vi "writeSettingsFile4ch.vi"(4 "delimiter (,)":string=",", 6 "message (overrides settings)":string, 7 "timestamp (current)":timestamp, 8 "error in (no error)":errorcluster, 9 "old settings":T3={"sampling"=1000, "coincidence_window"=10, "delay_A"=0, "delay_B"=0, "delay_C"=0, "delay_D"=0, "sleep_A"=0, "sleep_B"=0, "sleep_C"=0, "sleep_D"=0, "config_multiple_1"=0} {"config_multiple_1" items=["ABC"=224, "ABD"=208, "ACD"=176, "BCD"=112, "ABCD"=240]; "sleep_D" max=100 step=5; "sleep_C" max=100 step=5; "sleep_B" max=100 step=5; "sleep_A" max=100 step=5; "delay_D" max=100 step=5; "delay_C" max=100 step=5; "delay_B" max=100 step=5; "delay_A" max=100 step=5; "coincidence_window" min=5 max=10000 step=5; "sampling" items=["1ms"=1, "2ms"=2, "3ms"=3, "4ms"=4, "5ms"=5, "6ms"=6, "7ms"=7, "8ms"=8, "9ms"=9, "10ms"=10, "11ms"=11, "12ms"=12, "13ms"=13, "14ms"=14, "15ms"=15, "16ms"=16, "17ms"=17, "18ms"=18, "19ms"=19, "20ms"=20, "21ms"=21, "22ms"=22, "23ms"=23, "24ms"=24, "25ms"=25, "26ms"=26, "27ms"=27, "28ms"=28, "29ms"=29, "30ms"=30, "31ms"=31, "32ms"=32, "33ms"=33, "34ms"=34, "35ms"=35, "36ms"=36, "37ms"=37, "38ms"=38, "39ms"=39, "40ms"=40, "41ms"=41, "42ms"=42, "43ms"=43, "44ms"=44, "45ms"=45, "46ms"=46, "47ms"=47, "48ms"=48, "49ms"=49, "50ms"=50, "51ms"=51, "52ms"=52, "53ms"=53, "54ms"=54, "55ms"=55, "56ms"=56, "57ms"=57, "58ms"=58, "59ms"=59, "60ms"=60, "61ms"=61, "62ms"=62, "63ms"=63, "64ms"=64, "65ms"=65, "66ms"=66, "67ms"=67, "68ms"=68, "69ms"=69, "70ms"=70, "71ms"=71, "72ms"=72, "73ms"=73, "74ms"=74, "75ms"=75, "76ms"=76, "77ms"=77, "78ms"=78, "79ms"=79, "80ms"=80, "81ms"=81, "82ms"=82, "83ms"=83, "84ms"=84, "85ms"=85, "86ms"=86, "87ms"=87, "88ms"=88, "89ms"=89, "90ms"=90, "91ms"=91, "92ms"=92, "93ms"=93, "94ms"=94, "95ms"=95, "96ms"=96, "97ms"=97, "98ms"=98, "99ms"=99, "100ms"=100, "110ms"=110, "120ms"=120, "130ms"=130, "140ms"=140, "150ms"=150, "160ms"=160, "170ms"=170, "180ms"=180, "190ms"=190, "200ms"=200, "210ms"=210, "220ms"=220, "230ms"=230, "240ms"=240, "250ms"=250, "260ms"=260, "270ms"=270, "280ms"=280, "290ms"=290, "300ms"=300, "310ms"=310, "320ms"=320, "330ms"=330, "340ms"=340, "350ms"=350, "360ms"=360, "370ms"=370, "380ms"=380, "390ms"=390, "400ms"=400, "410ms"=410, "420ms"=420, "430ms"=430, "440ms"=440, "450ms"=450, "460ms"=460, "470ms"=470, "480ms"=480, "490ms"=490, "500ms"=500, "510ms"=510, "520ms"=520, "530ms"=530, "540ms"=540, "550ms"=550, "560ms"=560, "570ms"=570, "580ms"=580, "590ms"=590, "600ms"=600, "610ms"=610, "620ms"=620, "630ms"=630, "640ms"=640, "650ms"=650, "660ms"=660, "670ms"=670, "680ms"=680, "690ms"=690, "700ms"=700, "710ms"=710, "720ms"=720, "730ms"=730, "740ms"=740, "750ms"=750, "760ms"=760, "770ms"=770, "780ms"=780, "790ms"=790, "800ms"=800, "810ms"=810, "820ms"=820, "830ms"=830, "840ms"=840, "850ms"=850, "860ms"=860, "870ms"=870, "880ms"=880, "890ms"=890, "900ms"=900, "910ms"=910, "920ms"=920, "930ms"=930, "940ms"=940, "950ms"=950, "960ms"=960, "970ms"=970, "980ms"=980, "990ms"=990, "1,0s"=1000, "1,1s"=1100, "1,2s"=1200, "1,3s"=1300, "1,4s"=1400, "1,5s"=1500, "1,6s"=1600, "1,7s"=1700, "1,8s"=1800, "1,9s"=1900, "2,0s"=2000, "2,1s"=2100, "2,2s"=2200, "2,3s"=2300, "2,4s"=2400, "2,5s"=2500, "2,6s"=2600, "2,7s"=2700, "2,8s"=2800, "2,9s"=2900, "3,0s"=3000, "3,1s"=3100, "3,2s"=3200, "3,3s"=3300, "3,4s"=3400, "3,5s"=3500, "3,6s"=3600, "3,7s"=3700, "3,8s"=3800, "3,9s"=3900, "4,0s"=4000, "4,1s"=4100, "4,2s"=4200, "4,3s"=4300, "4,4s"=4400, "4,5s"=4500, "4,6s"=4600, "4,7s"=4700, "4,8s"=4800, "4,9s"=4900, "5,0s"=5000, "5,1s"=5100, "5,2s"=5200, "5,3s"=5300, "5,4s"=5400, "5,5s"=5500, "5,6s"=5600, "5,7s"=5700, "5,8s"=5800, "5,9s"=5900, "6,0s"=6000, "6,1s"=6100, "6,2s"=6200, "6,3s"=6300, "6,4s"=6400, "6,5s"=6500, "6,6s"=6600, "6,7s"=6700, "6,8s"=6800, "6,9s"=6900, "7,0s"=7000, "7,1s"=7100, "7,2s"=7200, "7,3s"=7300, "7,4s"=7400, "7,5s"=7500, "7,6s"=7600, "7,7s"=7700, "7,8s"=7800, "7,9s"=7900, "8,0s"=8000, "8,1s"=8100, "8,2s"=8200, "8,3s"=8300, "8,4s"=8400, "8,5s"=8500, "8,6s"=8600, "8,7s"=8700, "8,8s"=8800, "8,9s"=8900, "9,0s"=9000, "9,1s"=9100, "9,2s"=9200, "9,3s"=9300, "9,4s"=9400, "9,5s"=9500, "9,6s"=9600, "9,7s"=9700, "9,8s"=9800, "9,9s"=9900, "10s"=10000, "11s"=11000, "12s"=12000, "13s"=13000, "14s"=14000, "15s"=15000, "16s"=16000, "17s"=17000, "18s"=18000, "19s"=19000, "20s"=20000, "21s"=21000, "22s"=22000, "23s"=23000, "24s"=24000, "25s"=25000, "26s"=26000, "27s"=27000, "28s"=28000, "29s"=29000, "30s"=30000, "31s"=31000, "32s"=32000, "33s"=33000, "34s"=34000, "35s"=35000, "36s"=36000, "37s"=37000, "38s"=38000, "39s"=39000, "40s"=40000, "41s"=41000, "42s"=42000, "43s"=43000, "44s"=44000, "45s"=45000, "46s"=46000, "47s"=47000, "48s"=48000, "49s"=49000, "50s"=50000, "51s"=51000, "52s"=52000, "53s"=53000, "54s"=54000, "55s"=55000, "56s"=56000, "57s"=57000, "58s"=58000, "59s"=59000, "60s"=60000, "61s"=61000, "62s"=62000, "63s"=63000, "64s"=64000, "65s"=65000, "66s"=66000, "67s"=67000, "68s"=68000, "69s"=69000, "70s"=70000, "71s"=71000, "72s"=72000, "73s"=73000, "74s"=74000, "75s"=75000, "76s"=76000, "77s"=77000, "78s"=78000, "79s"=79000, "80s"=80000, "81s"=81000, "82s"=82000, "83s"=83000, "84s"=84000, "85s"=85000, "86s"=86000, "87s"=87000, "88s"=88000, "89s"=89000, "90s"=90000, "91s"=91000, "92s"=92000, "93s"=93000, "94s"=94000, "95s"=95000, "96s"=96000, "97s"=97000, "98s"=98000, "99s"=99000, "100s"=100000, "110s"=110000, "120s"=120000, "130s"=130000, "140s"=140000, "150s"=150000, "160s"=160000, "170s"=170000, "180s"=180000, "190s"=190000, "200s"=200000, "210s"=210000, "220s"=220000, "230s"=230000, "240s"=240000, "250s"=250000, "260s"=260000, "270s"=270000, "280s"=280000, "290s"=290000, "300s"=300000, "310s"=310000, "320s"=320000, "330s"=330000, "340s"=340000, "350s"=350000, "360s"=360000, "370s"=370000, "380s"=380000, "390s"=390000, "400s"=400000, "410s"=410000, "420s"=420000, "430s"=430000, "440s"=440000, "450s"=450000, "460s"=460000, "470s"=470000, "480s"=480000, "490s"=490000, "500s"=500000, "510s"=510000, "520s"=520000, "530s"=530000, "540s"=540000, "550s"=550000, "560s"=560000, "570s"=570000, "580s"=580000, "590s"=590000, "600s"=600000, "610s"=610000, "620s"=620000, "630s"=630000, "640s"=640000, "650s"=650000, "660s"=660000, "670s"=670000, "680s"=680000, "690s"=690000, "700s"=700000, "710s"=710000, "720s"=720000, "730s"=730000, "740s"=740000, "750s"=750000, "760s"=760000, "770s"=770000, "780s"=780000, "790s"=790000, "800s"=800000, "810s"=810000, "820s"=820000, "830s"=830000, "840s"=840000, "850s"=850000, "860s"=860000, "870s"=870000, "880s"=880000, "890s"=890000, "900s"=900000, "910s"=910000, "920s"=920000, "930s"=930000, "940s"=940000, "950s"=950000, "960s"=960000, "970s"=970000, "980s"=980000, "990s"=990000, "1000s"=1000000]}, 10 "new settings":T3={"sampling"=1000, "coincidence_window"=10, "delay_A"=0, "delay_B"=0, "delay_C"=0, "delay_D"=0, "sleep_A"=0, "sleep_B"=0, "sleep_C"=0, "sleep_D"=0, "config_multiple_1"=0} {"config_multiple_1" items=["ABC"=224, "ABD"=208, "ACD"=176, "BCD"=112, "ABCD"=240]; "sleep_D" max=100 step=5; "sleep_C" max=100 step=5; "sleep_B" max=100 step=5; "sleep_A" max=100 step=5; "delay_D" max=100 step=5; "delay_C" max=100 step=5; "delay_B" max=100 step=5; "delay_A" max=100 step=5; "coincidence_window" min=5 max=10000 step=5; "sampling" items=["1ms"=1, "2ms"=2, "3ms"=3, "4ms"=4, "5ms"=5, "6ms"=6, "7ms"=7, "8ms"=8, "9ms"=9, "10ms"=10, "11ms"=11, "12ms"=12, "13ms"=13, "14ms"=14, "15ms"=15, "16ms"=16, "17ms"=17, "18ms"=18, "19ms"=19, "20ms"=20, "21ms"=21, "22ms"=22, "23ms"=23, "24ms"=24, "25ms"=25, "26ms"=26, "27ms"=27, "28ms"=28, "29ms"=29, "30ms"=30, "31ms"=31, "32ms"=32, "33ms"=33, "34ms"=34, "35ms"=35, "36ms"=36, "37ms"=37, "38ms"=38, "39ms"=39, "40ms"=40, "41ms"=41, "42ms"=42, "43ms"=43, "44ms"=44, "45ms"=45, "46ms"=46, "47ms"=47, "48ms"=48, "49ms"=49, "50ms"=50, "51ms"=51, "52ms"=52, "53ms"=53, "54ms"=54, "55ms"=55, "56ms"=56, "57ms"=57, "58ms"=58, "59ms"=59, "60ms"=60, "61ms"=61, "62ms"=62, "63ms"=63, "64ms"=64, "65ms"=65, "66ms"=66, "67ms"=67, "68ms"=68, "69ms"=69, "70ms"=70, "71ms"=71, "72ms"=72, "73ms"=73, "74ms"=74, "75ms"=75, "76ms"=76, "77ms"=77, "78ms"=78, "79ms"=79, "80ms"=80, "81ms"=81, "82ms"=82, "83ms"=83, "84ms"=84, "85ms"=85, "86ms"=86, "87ms"=87, "88ms"=88, "89ms"=89, "90ms"=90, "91ms"=91, "92ms"=92, "93ms"=93, "94ms"=94, "95ms"=95, "96ms"=96, "97ms"=97, "98ms"=98, "99ms"=99, "100ms"=100, "110ms"=110, "120ms"=120, "130ms"=130, "140ms"=140, "150ms"=150, "160ms"=160, "170ms"=170, "180ms"=180, "190ms"=190, "200ms"=200, "210ms"=210, "220ms"=220, "230ms"=230, "240ms"=240, "250ms"=250, "260ms"=260, "270ms"=270, "280ms"=280, "290ms"=290, "300ms"=300, "310ms"=310, "320ms"=320, "330ms"=330, "340ms"=340, "350ms"=350, "360ms"=360, "370ms"=370, "380ms"=380, "390ms"=390, "400ms"=400, "410ms"=410, "420ms"=420, "430ms"=430, "440ms"=440, "450ms"=450, "460ms"=460, "470ms"=470, "480ms"=480, "490ms"=490, "500ms"=500, "510ms"=510, "520ms"=520, "530ms"=530, "540ms"=540, "550ms"=550, "560ms"=560, "570ms"=570, "580ms"=580, "590ms"=590, "600ms"=600, "610ms"=610, "620ms"=620, "630ms"=630, "640ms"=640, "650ms"=650, "660ms"=660, "670ms"=670, "680ms"=680, "690ms"=690, "700ms"=700, "710ms"=710, "720ms"=720, "730ms"=730, "740ms"=740, "750ms"=750, "760ms"=760, "770ms"=770, "780ms"=780, "790ms"=790, "800ms"=800, "810ms"=810, "820ms"=820, "830ms"=830, "840ms"=840, "850ms"=850, "860ms"=860, "870ms"=870, "880ms"=880, "890ms"=890, "900ms"=900, "910ms"=910, "920ms"=920, "930ms"=930, "940ms"=940, "950ms"=950, "960ms"=960, "970ms"=970, "980ms"=980, "990ms"=990, "1,0s"=1000, "1,1s"=1100, "1,2s"=1200, "1,3s"=1300, "1,4s"=1400, "1,5s"=1500, "1,6s"=1600, "1,7s"=1700, "1,8s"=1800, "1,9s"=1900, "2,0s"=2000, "2,1s"=2100, "2,2s"=2200, "2,3s"=2300, "2,4s"=2400, "2,5s"=2500, "2,6s"=2600, "2,7s"=2700, "2,8s"=2800, "2,9s"=2900, "3,0s"=3000, "3,1s"=3100, "3,2s"=3200, "3,3s"=3300, "3,4s"=3400, "3,5s"=3500, "3,6s"=3600, "3,7s"=3700, "3,8s"=3800, "3,9s"=3900, "4,0s"=4000, "4,1s"=4100, "4,2s"=4200, "4,3s"=4300, "4,4s"=4400, "4,5s"=4500, "4,6s"=4600, "4,7s"=4700, "4,8s"=4800, "4,9s"=4900, "5,0s"=5000, "5,1s"=5100, "5,2s"=5200, "5,3s"=5300, "5,4s"=5400, "5,5s"=5500, "5,6s"=5600, "5,7s"=5700, "5,8s"=5800, "5,9s"=5900, "6,0s"=6000, "6,1s"=6100, "6,2s"=6200, "6,3s"=6300, "6,4s"=6400, "6,5s"=6500, "6,6s"=6600, "6,7s"=6700, "6,8s"=6800, "6,9s"=6900, "7,0s"=7000, "7,1s"=7100, "7,2s"=7200, "7,3s"=7300, "7,4s"=7400, "7,5s"=7500, "7,6s"=7600, "7,7s"=7700, "7,8s"=7800, "7,9s"=7900, "8,0s"=8000, "8,1s"=8100, "8,2s"=8200, "8,3s"=8300, "8,4s"=8400, "8,5s"=8500, "8,6s"=8600, "8,7s"=8700, "8,8s"=8800, "8,9s"=8900, "9,0s"=9000, "9,1s"=9100, "9,2s"=9200, "9,3s"=9300, "9,4s"=9400, "9,5s"=9500, "9,6s"=9600, "9,7s"=9700, "9,8s"=9800, "9,9s"=9900, "10s"=10000, "11s"=11000, "12s"=12000, "13s"=13000, "14s"=14000, "15s"=15000, "16s"=16000, "17s"=17000, "18s"=18000, "19s"=19000, "20s"=20000, "21s"=21000, "22s"=22000, "23s"=23000, "24s"=24000, "25s"=25000, "26s"=26000, "27s"=27000, "28s"=28000, "29s"=29000, "30s"=30000, "31s"=31000, "32s"=32000, "33s"=33000, "34s"=34000, "35s"=35000, "36s"=36000, "37s"=37000, "38s"=38000, "39s"=39000, "40s"=40000, "41s"=41000, "42s"=42000, "43s"=43000, "44s"=44000, "45s"=45000, "46s"=46000, "47s"=47000, "48s"=48000, "49s"=49000, "50s"=50000, "51s"=51000, "52s"=52000, "53s"=53000, "54s"=54000, "55s"=55000, "56s"=56000, "57s"=57000, "58s"=58000, "59s"=59000, "60s"=60000, "61s"=61000, "62s"=62000, "63s"=63000, "64s"=64000, "65s"=65000, "66s"=66000, "67s"=67000, "68s"=68000, "69s"=69000, "70s"=70000, "71s"=71000, "72s"=72000, "73s"=73000, "74s"=74000, "75s"=75000, "76s"=76000, "77s"=77000, "78s"=78000, "79s"=79000, "80s"=80000, "81s"=81000, "82s"=82000, "83s"=83000, "84s"=84000, "85s"=85000, "86s"=86000, "87s"=87000, "88s"=88000, "89s"=89000, "90s"=90000, "91s"=91000, "92s"=92000, "93s"=93000, "94s"=94000, "95s"=95000, "96s"=96000, "97s"=97000, "98s"=98000, "99s"=99000, "100s"=100000, "110s"=110000, "120s"=120000, "130s"=130000, "140s"=140000, "150s"=150000, "160s"=160000, "170s"=170000, "180s"=180000, "190s"=190000, "200s"=200000, "210s"=210000, "220s"=220000, "230s"=230000, "240s"=240000, "250s"=250000, "260s"=260000, "270s"=270000, "280s"=280000, "290s"=290000, "300s"=300000, "310s"=310000, "320s"=320000, "330s"=330000, "340s"=340000, "350s"=350000, "360s"=360000, "370s"=370000, "380s"=380000, "390s"=390000, "400s"=400000, "410s"=410000, "420s"=420000, "430s"=430000, "440s"=440000, "450s"=450000, "460s"=460000, "470s"=470000, "480s"=480000, "490s"=490000, "500s"=500000, "510s"=510000, "520s"=520000, "530s"=530000, "540s"=540000, "550s"=550000, "560s"=560000, "570s"=570000, "580s"=580000, "590s"=590000, "600s"=600000, "610s"=610000, "620s"=620000, "630s"=630000, "640s"=640000, "650s"=650000, "660s"=660000, "670s"=670000, "680s"=680000, "690s"=690000, "700s"=700000, "710s"=710000, "720s"=720000, "730s"=730000, "740s"=740000, "750s"=750000, "760s"=760000, "770s"=770000, "780s"=780000, "790s"=790000, "800s"=800000, "810s"=810000, "820s"=820000, "830s"=830000, "840s"=840000, "850s"=850000, "860s"=860000, "870s"=870000, "880s"=880000, "890s"=890000, "900s"=900000, "910s"=910000, "920s"=920000, "930s"=930000, "940s"=940000, "950s"=950000, "960s"=960000, "970s"=970000, "980s"=980000, "990s"=990000, "1000s"=1000000]}, 11 "path":path) -> (0 "error out":errorcluster, 2 "text written":string[][](array[string]))   [LabVIEW 2015]
doc: "If a string is given at the 'message' input, writes it into the file with a timestamp in the format:\n timestamp, message \nElse, writes into the specified file each of the given 'new settings' that has changed compared to the 'old settings'. Includes a timestamp, in the format:\n timestamp, setting, value+units."
uses:
  <instrlib>/Tausand AB1000/Public/Controls/settings4ch.ctl
  <instrlib>/Tausand AB1000/Public/Controls/configMultipleCoincRing.ctl
  <vilib>/Utility/file.llb/Write Delimited Spreadsheet (string).vi
  <instrlib>/Tausand AB1000/Tausand AB1000.lvlib
panel:
  out "change in settings?":T1
  in  "config_multiple":T2 caption="Config. multiple" items=["ABC"=224, "ABD"=208, "ABE"=200, "ABF"=196, "ABG"=194, "ABH"=193, "ACD"=176, "ACE"=168, "ACF"=164, "ACG"=162, "ACH"=161, "ADE"=152, "ADF"=148, "ADG"=146, "ADH"=145, "AEF"=140, "AEG"=138, "AEH"=137, "AFG"=134, "AFH"=133, "AGH"=131, "BCD"=112, "BCE"=104, "BCF"=100, "BCG"=98, "BCH"=97, "BDE"=88, "BDF"=84, "BDG"=82, "BDH"=81, "BEF"=76, "BEG"=74, "BEH"=73, "BFG"=70, "BFH"=69, "BGH"=67, "CDE"=56, "CDF"=52, "CDG"=50, "CDH"=49, "CEF"=44, "CEG"=42, "CEH"=41, "CFG"=38, "CFH"=37, "CGH"=35, "DEF"=28, "DEG"=26, "DEH"=25, "DFG"=22, "DFH"=21, "DGH"=19, "EFG"=14, "EFH"=13, "EGH"=11, "FGH"=7, "ABCD"=240, "ABCE"=232, "ABCF"=228, "ABCG"=226, "ABCH"=225, "ABDE"=216, "ABDF"=212, "ABDG"=210, "ABDH"=209, "ABEF"=204, "ABEG"=202, "ABEH"=201, "ABFG"=198, "ABFH"=197, "ABGH"=195, "ACDE"=184, "ACDF"=180, "ACDG"=178, "ACDH"=177, "ACEF"=172, "ACEG"=170, "ACEH"=169, "ACFG"=166, "ACFH"=165, "ACGH"=163, "ADEF"=156, "ADEG"=154, "ADEH"=153, "ADFG"=150, "ADFH"=149, "ADGH"=147, "AEFG"=142, "AEFH"=141, "AEGH"=139, "AFGH"=135, "BCDE"=120, "BCDF"=116, "BCDG"=114, "BCDH"=113, "BCEF"=108, "BCEG"=106, "BCEH"=105, "BCFG"=102, "BCFH"=101, "BCGH"=99, "BDEF"=92, "BDEG"=90, "BDEH"=89, "BDFG"=86, "BDFH"=85, "BDGH"=83, "BEFG"=78, "BEFH"=77, "BEGH"=75, "BFGH"=71, "CDEF"=60, "CDEG"=58, "CDEH"=57, "CDFG"=54, "CDFH"=53, "CDGH"=51, "CEFG"=46, "CEFH"=45, "CEGH"=43, "CFGH"=39, "DEFG"=30, "DEFH"=29, "DEGH"=27, "DFGH"=23, "EFGH"=15]
  out "use current timestamp?":bool
  out "setting unit":string[](array[string])
  out "setting value":u32[](array[numeric])
  out "setting name":string[](array[string])
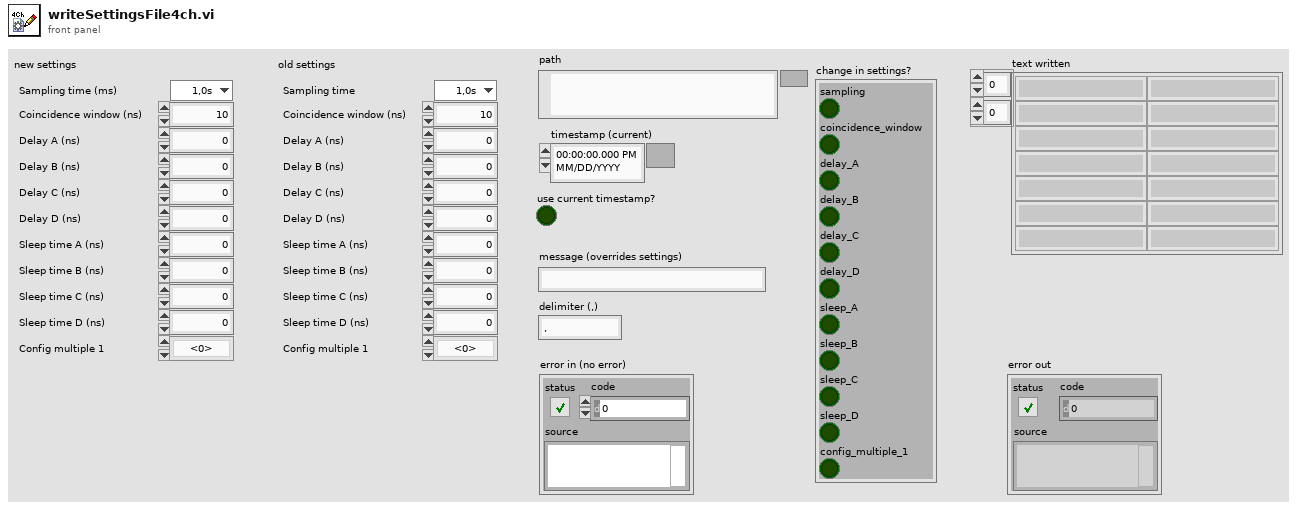
[diagram p1: front panel]
types:
  T1 = cluster{"sampling":bool, "coincidence_window":bool, "delay_A":bool, "delay_B":bool, "delay_C":bool, "delay_D":bool, "sleep_A":bool, "sleep_B":bool, "sleep_C":bool, "sleep_D":bool, "config_multiple_1":bool}
  T2 = typedef "Tausand AB1000.lvlib/configMultipleCoincRing.ctl" = u16
  T3 = typedef "Tausand AB1000.lvlib/settings4ch.ctl" = cluster{"sampling":u32, "coincidence_window":u32, "delay_A":u32, "delay_B":u32, "delay_C":u32, "delay_D":u32, "sleep_A":u32, "sleep_B":u32, "sleep_C":u32, "sleep_D":u32, "config_multiple_1":T2}
  T4 = typedef "LVStringsAndValuesArrayTypeDef_U16.ctl" = cluster{"String":string, "Value":u16}[]
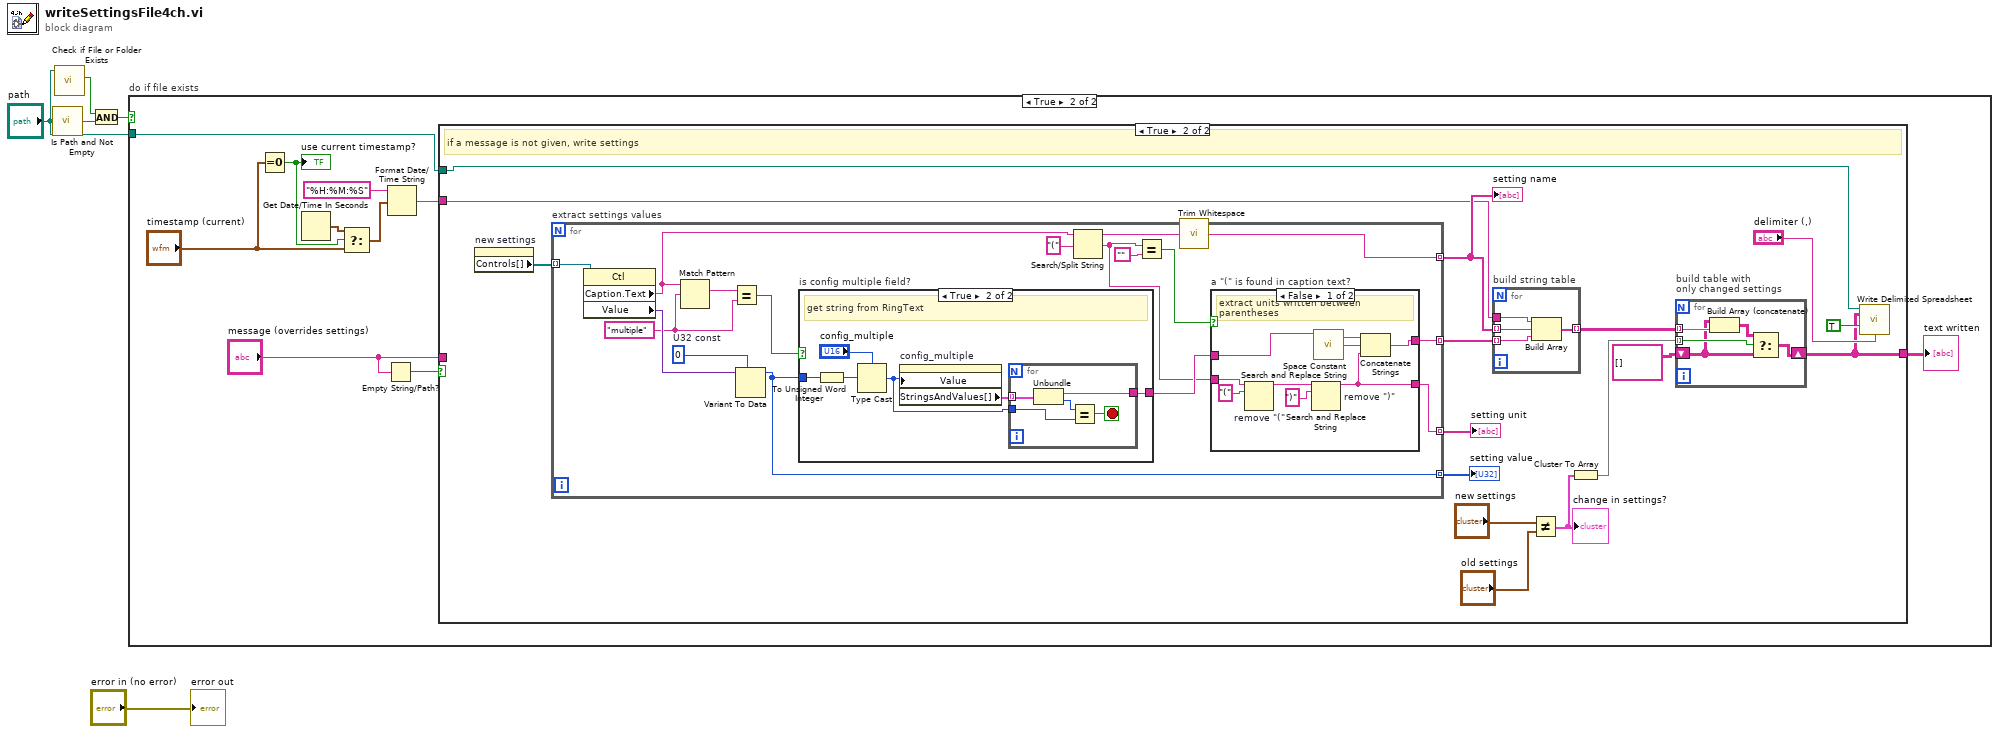
[diagram p0: block diagram]
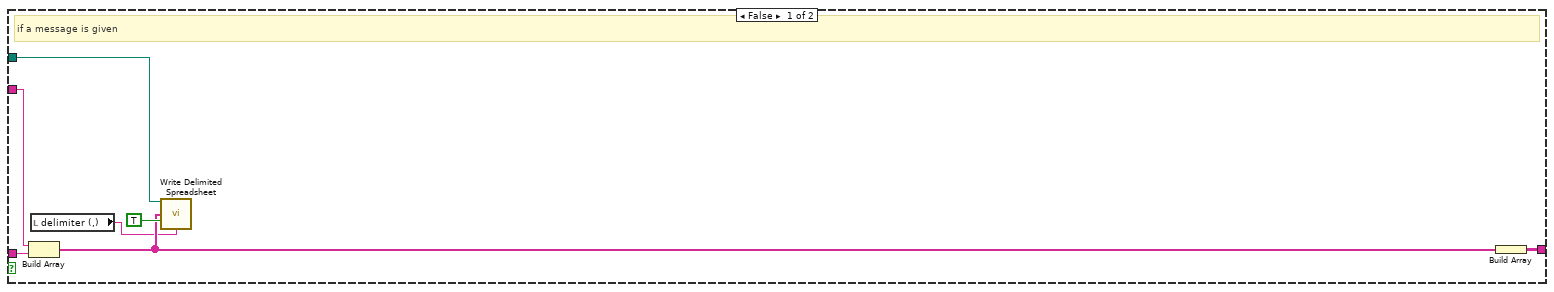
[diagram p3: hidden frame]
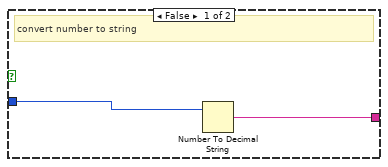
[diagram p4: hidden frame]
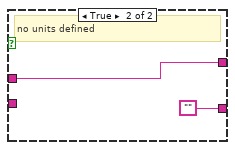
[diagram p5: hidden frame]
diagram:
  n1 = call <vilib>:"Is Path and Not Empty.vi"("path"="path") -> ("Is Path and Not Empty?"=w4:bool)  [unwired: 4 in]
  n2 = call <vilib>:"Check if File or Folder Exists.vi"("path"="path") -> ("file or folder exists?"=w3:bool)  [unwired: 8 in, 2 out]
  n3 = And(x=w3, y=w4) -> (x .and. y?=w2:bool)
  n4 = case "do if file exists" shown="True" w2 {
    tunnel: "path" -> [_ w13]
    frame False {
    }
    frame True {
      n5 = Equal To 0?(x="timestamp (current)") -> (x = 0?=w12:bool)
      "use current timestamp?" <- w12
      n6 = Get Date/Time In Seconds() -> (seconds since 1Jan1904=w10:timestamp)
      n7 = Select(t=w10, s=w12, f="timestamp (current)") -> (s? t:f=w9:timestamp)
      n8 = Empty String/Path?(string/path="message (overrides settings)") -> (empty?=w15:bool)
      n9 = Format Date/Time String(time format string (%c)="%H:%M:%S", seconds (now)=w9) -> (date/time string=w7:string)  [unwired: 1 in]
      n10 = case shown="True" w15 {
        tunnel: "message (overrides settings)" -> [w19 _]
        tunnel: w7 -> [w20 w36]
        tunnel: w13 -> [w21 w35]
        tunnel: [w17 w27] -> w6
        frame False {
          # "if a message is given"
          n11 = Build Array(w20, w19) -> (w18:string[])
          n12 = local read "delimiter (,)"() -> (w16:string)
          n13 = call-poly <vilib>:"Write Delimited Spreadsheet.vi"("file path (dialog if empty)"=w21, "1D data"=w18, "append to file? (F)"=TRUE, "delimiter (\\t)"=w16) -> ()  [unwired: 10 in, 2 out]
          n14 = Build Array(w18) -> (w17:string[][])
        }
        frame True {
          # "if a message is not given, write settings"
          n15 = property on="new settings" class="Clust (strict)"() -> ("Controls[]"=w26:refnum<vi>[])  [unwired: 2 in, 2 out]
          n16 = for "extract settings values" {
            tunnel: w26 -> [w55] mode=indexing
            tunnel: [w47] -> w37 mode=indexing
            tunnel: [w50] -> w38 mode=indexing
            tunnel: [w41] -> w24 mode=indexing
            tunnel: [w40] -> w23 mode=indexing
            w46 = "multiple" ("regular expression")
            w53 = u32 0  # U32 const
            n17 = property class="Ctl"(reference=w55) -> ("Caption.Text"=w49:string, "Value"=w54:variant)  [unwired: 1 in, 2 out]
            n18 = Match Pattern(string=w49, regular expression=w46) -> (match substring=w45:string)  [unwired: 1 in, 3 out]
            n19 = Equal?(x=w45, y=w46) -> (x = y?=w48:bool)
            n20 = Variant To Data(type=w53, Variant=w54) -> (data=w47:u32)  [unwired: 1 in, 1 out]
            n21 = case "is config multiple field?" shown="True" w48 {
              tunnel: w47 -> [w57 w59]
              tunnel: [w56 w63] -> w42
              frame False {
                # "convert number to string"
                n22 = Number To Decimal String(number=w57) -> (decimal integer string=w56:string)  [unwired: 1 in]
              }
              frame True {
                # "get string from RingText"
                n23 = To Unsigned Word Integer(number=w59) -> (unsigned 16bit integer=w58:u16)
                n24 = Type Cast(type="config_multiple", x=w58) -> (*(type *) &x=w60:T2)
                n25 = property on="config_multiple" class="Ring (strict)"("Value"=w60) -> ("StringsAndValues[]"=w62:T4)  [unwired: 2 in, 2 out]
                n26 = for {
                  tunnel: w62 -> [w68] mode=indexing
                  tunnel: w60 -> [w66]
                  tunnel: [w64] -> w63
                  stop <- w65 stop-if-true
                  n27 = Unbundle(w68) -> ("String"=w64:string, "Value"=w67:u16)
                  n28 = Equal?(x=w67, y=w66) -> (x = y?=w65:bool)
                }
              }
            }
            n29 = Search/Split String(string=w49, search string/char (-)="(") -> (substring before match=w51:string, match + rest of string=w39:string)  [unwired: 1 in, 1 out]
            n30 = Equal?(x=w39, y="") -> (x = y?=w43:bool)
            n31 = call <vilib>:"Trim Whitespace.vi"("string"=w51) -> ("trimmed string"=w50:string)  [unwired: 1 in]
            n32 = case "a \"(\" is found in caption text?" shown="False" w43 {
              tunnel: [w72 w78] -> w41
              tunnel: w42 -> [w71 w78]
              tunnel: [w70 "" ("result string")] -> w40
              tunnel: w39 -> [w69 _]
              frame False {
                # "extract units written between parentheses"
                n33 = Search and Replace String "remove \"(\""(input string=w69, search string="(" ("search string/char (-)")) -> (result string=w76:string)  [unwired: 6 in, 3 out]
                n34 = Search and Replace String "remove \")\""(input string=w76, search string=")" ("search string/char (-)")) -> (result string=w70:string)  [unwired: 6 in, 3 out]
                n35 = call <vilib>:"Space Constant.vi"() -> ("String"=w73:string)
                n36 = Concatenate Strings(w71, w73, w70) -> (w72:string)
              }
              frame True {
                # "no units defined"
              }
            }
          }
          "setting name" <- w38
          "setting value" <- w37
          "setting unit" <- w23
          n37 = for "build string table" {
            tunnel: w38 -> [w87] mode=indexing
            tunnel: [w86] -> w29 mode=indexing
            tunnel: w36 -> [w85]
            tunnel: w24 -> [w84] mode=indexing
            n38 = Build Array(w85, w87, w84) -> (w86:string[])
          }
          n39 = Not Equal?(x="new settings", y="old settings") -> (x != y?=w25:T1)
          "change in settings?" <- w25
          n40 = Cluster To Array(cluster=w25) -> (array=w30:bool[])
          n41 = for "build table with\nonly changed settings" {
            tunnel: w30 -> [w83] mode=indexing
            tunnel: w29 -> [w82] mode=indexing
            shift-right: [w80] -> w27
            shift-left: string[][] [] ("f") -> [w79]
            n42 = Build Array (concatenate)(w79, w82) -> (w81:string[][])
            n43 = Select(t=w81, s=w83, f=w79) -> (s? t:f=w80:string[][])
          }
          n44 = call-poly <vilib>:"Write Delimited Spreadsheet.vi"("file path (dialog if empty)"=w35, "2D data"=w27, "append to file? (F)"=TRUE, "delimiter (\\t)"="delimiter (,)") -> ()  [unwired: 10 in, 2 out]
        }
      }
      "text written" <- w6
    }
  }
  "error out" <- "error in (no error)"
